vi "Run Test.vi"(8 "error in (no error)":errorcluster, 11 "Plugin_UI in":refnum<class "Plugin_UI.lvclass">) -> (0 "error out":errorcluster, 2 "Plugin_Controller out":refnum<class "Plugin_Controller.lvclass">, 3 "Plugin_UI out":refnum<class "Plugin_UI.lvclass">)   [LabVIEW 2020, in "Plugin.lvlib" / "Plugin_UI.lvclass"]
doc: "Performs a quick test."
uses:
  Plugin_UI.lvclass
  Controller_Class/Plugin_Controller.lvclass
  Plugin_UI.lvclass/Plugin_UI.ctl
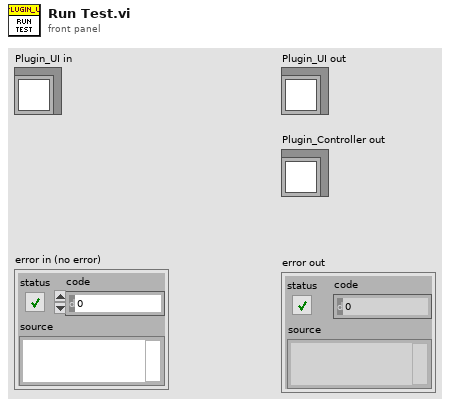
[diagram p1: front panel]
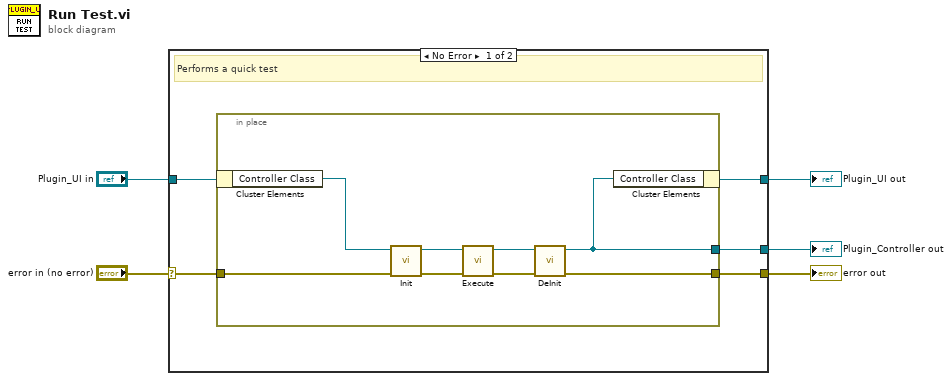
[diagram p0: block diagram]
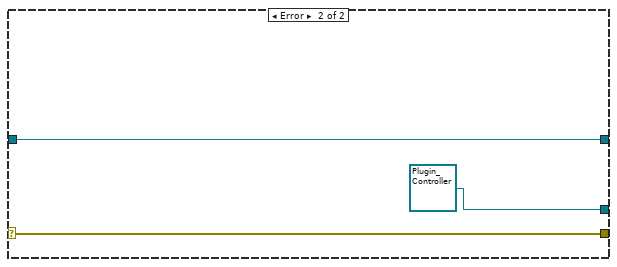
[diagram p2: hidden frame]
diagram:
  n1 = case shown="No Error" "error in (no error)" {
    selector: "error in (no error)" -> [w8 w20]
    tunnel: [w6 w21] -> w5
    tunnel: "Plugin_UI in" -> [w7 w21]
    tunnel: [w10 refnum<class "Plugin_Controller.lvclass"> refnum ("Plugin_Controller out")] -> w3
    tunnel: [w9 w20] -> w1
    frame No Error {
      # "Performs a quick test"
      n2 = in-place "In Place Element Structure" {
        in-place-border: [w14] -> w10
        in-place-border: [w13] -> w9
        in-place-border: w8 -> [w12]
        n3 = in-place-cluster #1(w7) -> ("Controller Class"=w11:refnum<class "Plugin_Controller.lvclass">)
        n4 = call-dynamic "Init.vi"("error in"=w12, "Plugin_Controller in"=w11) -> ("error out"=w18:errorcluster, "Plugin_Controller out"=w17:refnum<class "Plugin_Controller.lvclass">)  [unwired: 8 in]
        n5 = call-dynamic "Execute.vi"("error in"=w18, "Plugin_Controller in"=w17) -> ("error out"=w15:errorcluster, "Plugin_Controller out"=w16:refnum<class "Plugin_Controller.lvclass">)  [unwired: 8 in]
        n6 = call-dynamic "DeInit.vi"("error in"=w15, "Plugin_Controller in"=w16) -> ("error out"=w13:errorcluster, "Plugin_Controller out"=w14:refnum<class "Plugin_Controller.lvclass">)  [unwired: 8 in]
        n7 = in-place-cluster #1("Controller Class"=w14) -> (w6:refnum<class "Plugin_UI.lvclass">)
      }
    }
    frame Error {
    }
  }
  "Plugin_UI out" <- w5
  "Plugin_Controller out" <- w3
  "error out" <- w1
